vi "Receive Value Change Event.vi"(8 "error in (no error)":errorcluster, 10 "ValueChangeMsg":refnum<class "ValueChangeMsg.lvclass">, 11 "PauseResumeButtons In":refnum<class "PauseResumeButtons.lvclass">) -> (0 "error out":errorcluster, 3 "PauseResumeButtons Out":refnum<class "PauseResumeButtons.lvclass">)   [LabVIEW 2015, in "MVAExamples.lvlib" / "PauseResumeButtons.lvclass"]
doc: "<License>\nCopyright © 2017 Composed Systems, LLC | All rights reserved\nwww.composed.io\n\nAuthor: Ethan Stern <ethan.stern@composed.io>\n\nThis software is provided \"AS IS\" WITHOUT WARRANTIES, either express or implied, AND IS FOR EDUCATIONAL PURPOSES ONLY.\n</License>"
uses:
  PauseResumeButtons.lvclass
  Framework/ActorEvents/IEventAggregator Messages/ValueChangeMsg/ValueChangeMsg.lvclass
  Framework/ActorEvents/IEventAggregator Messages/ValueChangeMsg/ValueChangeMsg.lvclass/ValueChangeMsg.ctl
  PauseResumeButtons.lvclass/PauseResumeButtons.ctl
  Framework/ActorEvents/IEventAggregator Messages/ValueChangeMsg/Accessors/Read Control Label.vi
  Framework/IViewable/IViewable/IViewable.lvclass
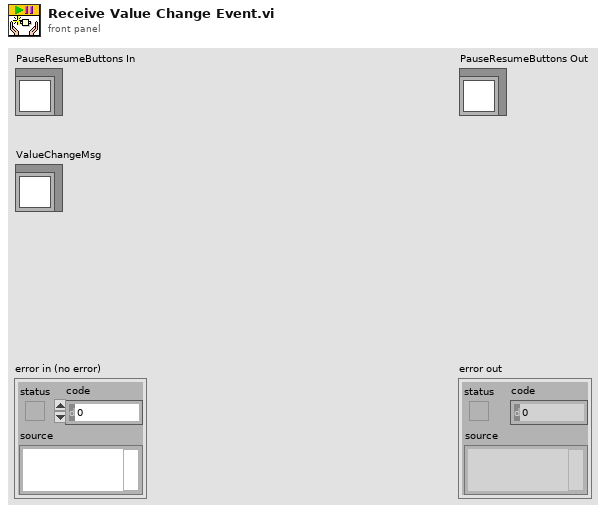
[diagram p1: front panel]
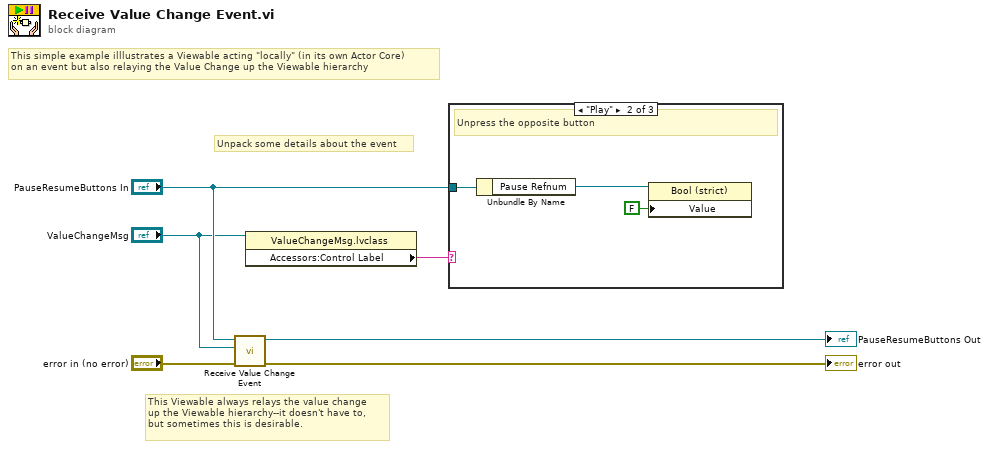
[diagram p0: block diagram]
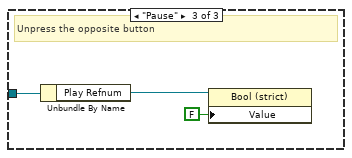
[diagram p3: hidden frame]
diagram:
  # "This simple example illlustrates a Viewable acting \"locally\" (in its own Actor Core)\non an event but also relaying the Value Change up the Viewable hierarchy"
  # "Unpack some details about the event"
  # "This Viewable always relays the value change\nup the Viewable hierarchy--it doesn't have to,\nbut sometimes this is desirable."
  n1 = call-parent "Receive Value Change Event.vi"("error in (no error)"="error in (no error)", "ValueChangeMsg"="ValueChangeMsg", "IViewable In"="PauseResumeButtons In") -> ("error out"=→"error out":errorcluster, "IViewable Out"=→"PauseResumeButtons Out":refnum<class "PauseResumeButtons.lvclass">)  [unwired: 7 in]
  n2 = property class="ValueChangeMsg.lvclass"(reference="ValueChangeMsg") -> ("Accessors:Control Label"=w1:string)  [unwired: 1 in, 2 out]
  n3 = case shown="\"Play\"" w1 {
    tunnel: "PauseResumeButtons In" -> [_ w9 w12]
    frame Default {
      # "Do nothing for unkown control"
    }
    frame "Play" {
      # "Unpress the opposite button"
      n4 = Unbundle By Name(w9) -> ("Pause Refnum"=w8:refnum<vi>)
      n5 = property class="Bool (strict)"(reference=w8, "Value"=FALSE) -> ()  [unwired: 1 in, 2 out]
    }
    frame "Pause" {
      # "Unpress the opposite button"
      n6 = Unbundle By Name(w12) -> ("Play Refnum"=w11:refnum<vi>)
      n7 = property class="Bool (strict)"(reference=w11, "Value"=FALSE) -> ()  [unwired: 1 in, 2 out]
    }
  }
